vi "Send CMD_M1.vi"(5 "Speed (mm/s) M1":i32, 6 "SERVO ON CMD M1":bool, 8 "Home Calling M1":bool, 9 "Pokayoka":bool, 10 "Travel (mm)M1":i32, 11 "Slide Servo":T1) -> ()   [LabVIEW 2015]
uses:
  Galobal variable_TI.vi
  Project Setup/Globle Variable/GR_Servo.vi
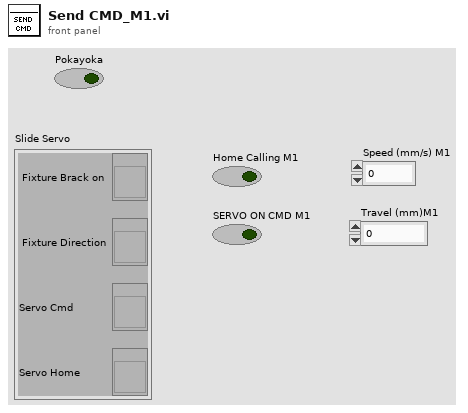
[diagram p1: front panel]
types:
  T1 = cluster{" Fixture Brack on":refnum<vi>, " Fixture Direction":refnum<vi>, "Servo Cmd":refnum<vi>, "Servo Home":refnum<vi>}
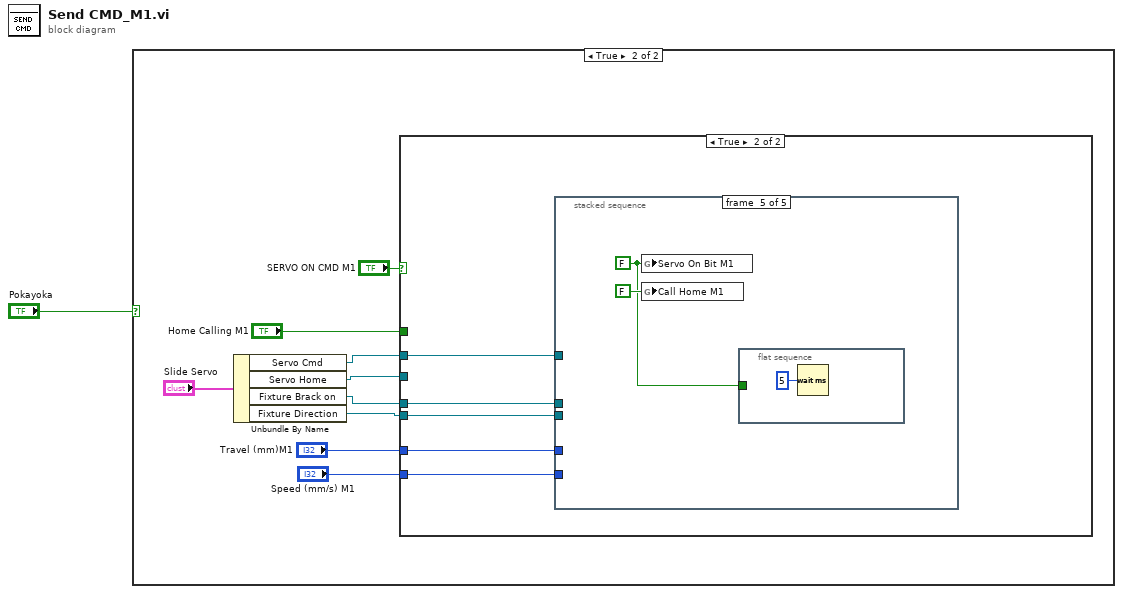
[diagram p0: block diagram]
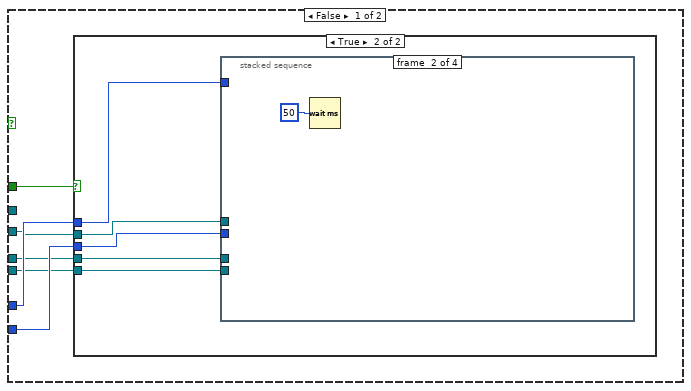
[diagram p3: hidden frame]
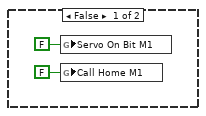
[diagram p4: hidden frame]
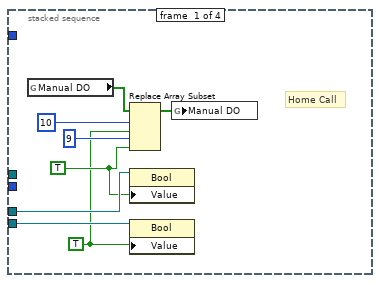
[diagram p5: hidden frame]
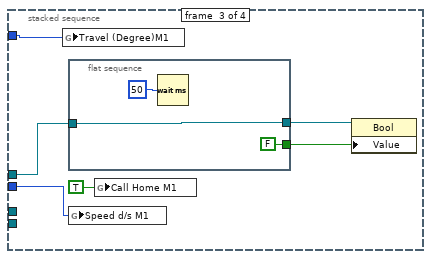
[diagram p6: hidden frame]
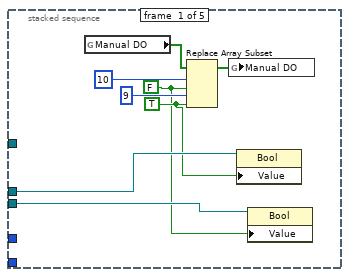
[diagram p8: hidden frame]
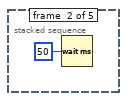
[diagram p9: hidden frame]
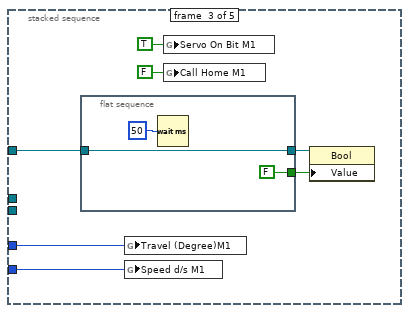
[diagram p10: hidden frame]
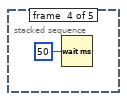
[diagram p11: hidden frame]
diagram:
  n1 = case shown="True" "Pokayoka" {
    frame False {
    }
    frame True {
      n2 = Unbundle By Name("Slide Servo") -> ("Servo Cmd"=w2:refnum<vi>, "Servo Home"=w3:refnum<vi>, "Fixture Brack on"=w5:refnum<vi>, "Fixture Direction"=w4:refnum<vi>)
      n3 = case shown="True" "SERVO ON CMD M1" {
        tunnel: "Speed (mm/s) M1" -> [w15 w46]
        tunnel: "Travel (mm)M1" -> [w14 w45]
        tunnel: "Home Calling M1" -> [w16 _]
        tunnel: w2 -> [_ w44]
        tunnel: w3 -> [w13 _]
        tunnel: w5 -> [w12 w43]
        tunnel: w4 -> [w11 w42]
        frame False {
          n4 = case shown="True" w16 {
            tunnel: w15 -> [_ w20]
            tunnel: w14 -> [_ w19]
            tunnel: w13 -> [_ w21]
            tunnel: w12 -> [_ w23]
            tunnel: w11 -> [_ w22]
            frame False {
              n5 = global write "GR_Servo.vi" "Servo On Bit M1"(FALSE ("Servo On Bit")) -> ()
              n6 = global write "Galobal variable_TI.vi" "Call Home M1"(FALSE ("Call Home M1")) -> ()
            }
            frame True {
              n7 = stacked-sequence {
                tunnel: w23 -> [w29 _ _ _]
                tunnel: w22 -> [w28 _ _ _]
                tunnel: w21 -> [_ _ w34 _]
                tunnel: w20 -> [_ _ w36 _]
                tunnel: w19 -> [_ _ w35 _]
                frame #0 {
                  w25 = TRUE ("new element/subarray")
                  w24 = TRUE ("new element/subarray")
                  # "Home Call"
                  n8 = global read "Galobal variable_TI.vi" "Manual DO"() -> (w26:bool[])
                  n9 = Replace Array Subset(array=w26, new element #1=w24, index #1=10 ("index"), new element #2=w25, index #2=9 ("index")) -> (w31:bool[])
                  n10 = property class="Bool"(reference=w29, "Value"=w25) -> ()  [unwired: 1 in, 2 out]
                  n11 = property class="Bool"(reference=w28, "Value"=w24) -> ()  [unwired: 1 in, 2 out]
                  n12 = global write "Galobal variable_TI.vi" "Manual DO"(w31) -> ()
                }
                frame #1 {
                  n13 = Wait (ms)(milliseconds to wait=u32 50) -> ()  [unwired: 1 out]
                }
                frame #2 {
                  n14 = global write "GR_Servo.vi" "Travel (Degree)M1"(w35) -> ()
                  n15 = flat-sequence {
                    tunnel: [FALSE ("SERVO ON CMD M1")] -> w37
                    tunnel: [w39] -> w33
                    tunnel: w34 -> [w39]
                    frame #0 {
                      n16 = Wait (ms)(milliseconds to wait=u32 50) -> ()  [unwired: 1 out]
                    }
                  }
                  n17 = global write "GR_Servo.vi" "Speed d/s M1"(w36) -> ()
                  n18 = global write "Galobal variable_TI.vi" "Call Home M1"(TRUE ("Call Home M1")) -> ()
                  n19 = property class="Bool"(reference=w33, "Value"=w37) -> ()  [unwired: 1 in, 2 out]
                }
                frame #3 {
                }
              }
            }
          }
        }
        frame True {
          n20 = stacked-sequence {
            tunnel: w46 -> [_ _ w62 _ _]
            tunnel: w45 -> [_ _ w61 _ _]
            tunnel: w44 -> [_ _ w58 _ _]
            tunnel: w43 -> [w50 _ _ _ _]
            tunnel: w42 -> [w49 _ _ _ _]
            frame #0 {
              w48 = TRUE ("new element/subarray")
              w47 = FALSE ("new element/subarray")
              n21 = global read "Galobal variable_TI.vi" "Manual DO"() -> (w51:bool[])
              n22 = Replace Array Subset(array=w51, new element #1=w47, index #1=10 ("index"), new element #2=w48, index #2=9 ("index")) -> (w54:bool[])
              n23 = global write "Galobal variable_TI.vi" "Manual DO"(w54) -> ()
              n24 = property class="Bool"(reference=w50, "Value"=w48) -> ()  [unwired: 1 in, 2 out]
              n25 = property class="Bool"(reference=w49, "Value"=w47) -> ()  [unwired: 1 in, 2 out]
            }
            frame #1 {
              n26 = Wait (ms)(milliseconds to wait=u32 50) -> ()  [unwired: 1 out]
            }
            frame #2 {
              n27 = flat-sequence {
                tunnel: [w64] -> w57
                tunnel: w58 -> [w64]
                tunnel: [FALSE ("SERVO ON CMD M1")] -> w56
                frame #0 {
                  n28 = Wait (ms)(milliseconds to wait=u32 50) -> ()  [unwired: 1 out]
                }
              }
              n29 = global write "GR_Servo.vi" "Travel (Degree)M1"(w61) -> ()
              n30 = global write "GR_Servo.vi" "Speed d/s M1"(w62) -> ()
              n31 = global write "GR_Servo.vi" "Servo On Bit M1"(TRUE ("Servo On Bit")) -> ()
              n32 = global write "Galobal variable_TI.vi" "Call Home M1"(FALSE ("Call Home M1")) -> ()
              n33 = property class="Bool"(reference=w57, "Value"=w56) -> ()  [unwired: 1 in, 2 out]
            }
            frame #3 {
              n34 = Wait (ms)(milliseconds to wait=u32 50) -> ()  [unwired: 1 out]
            }
            frame #4 {
              w67 = FALSE ("Servo On Bit")
              n35 = global write "GR_Servo.vi" "Servo On Bit M1"(w67) -> ()
              n36 = global write "Galobal variable_TI.vi" "Call Home M1"(FALSE ("Call Home M1")) -> ()
              n37 = flat-sequence {
                tunnel: w67 -> [_]
                frame #0 {
                  n38 = Wait (ms)(milliseconds to wait=u32 5) -> ()  [unwired: 1 out]
                }
              }
            }
          }
        }
      }
    }
  }
